vi "main.vi"() -> ()   [LabVIEW 2018]
uses:
  global.vi
  <vilib>/Utility/file.llb/Write Delimited Spreadsheet (string).vi
  <vilib>/Analysis/NI_AALBase.lvlib
panel:
  in  "开始测试":T1
  out "stimulus setup":T2
  in  "字符串":string
  out "二维图片":picture
  out "传声器 1":dbl[](graph)
  out "传声器 2":dbl[](graph)
  out "传声器 3":dbl[](graph)
  out "传声器 4":dbl[](graph)
  in  "阻抗测试绘图数据选择":u16(ring) items=["阻抗Z", "速度V"]
  in  "平滑":dbl(slide) scale=0.0..1.0
  out "速度V":cluster{"f":dbl[], dbl[]}[](graph)
  out "阻抗Z":cluster{dbl[], dbl[]}[](graph)
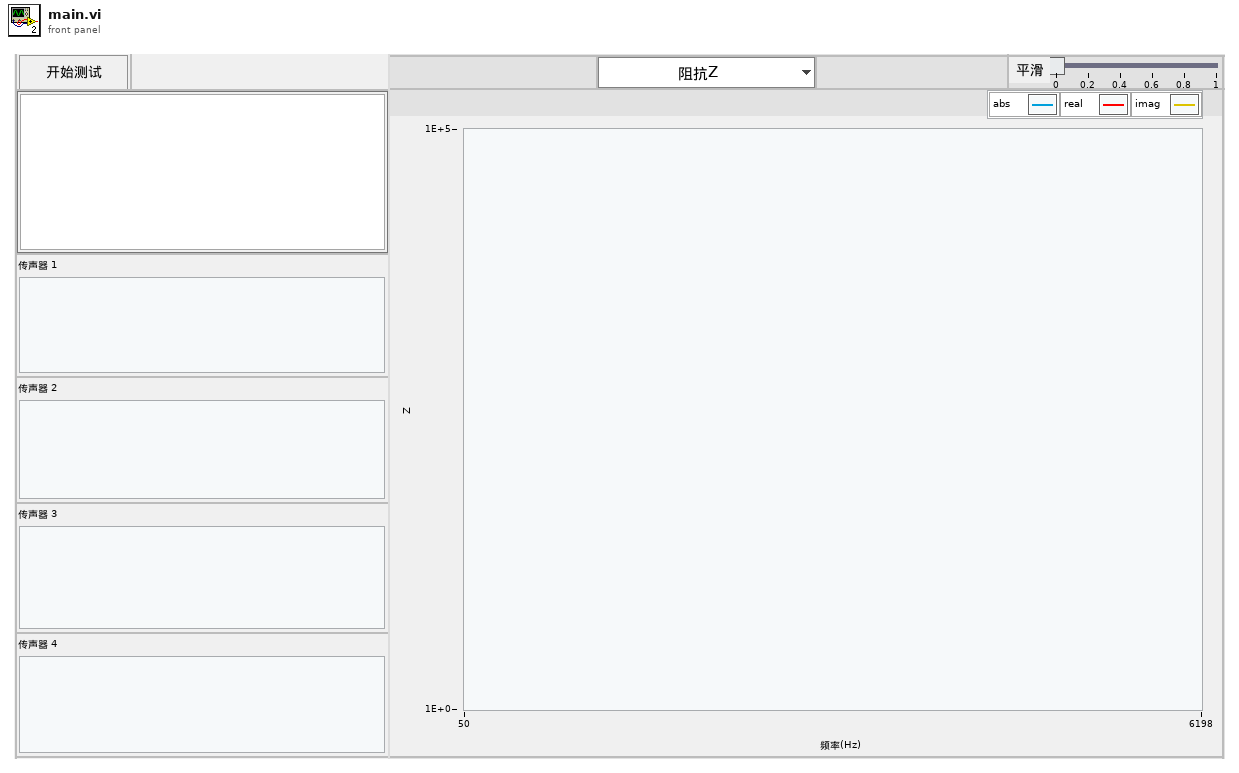
[diagram p1: front panel]
types:
  T1 = typedef "布尔控件.ctl" = bool
  T2 = cluster{"幅值(V)":dbl, "信号时长(s)":dbl, "频率上限(Hz)":dbl, "频率下限(Hz)":dbl}
  T3 = cluster{"f":dbl[], "传输阻抗Z":cdb[], "V":cdb[], "f_V":dbl[]}
  T4 = cluster{"管中温度：":dbl, "阻抗管内径d[mm]：":dbl, "传声器4到样品距离L[mm]：":dbl, "待测样品面积S[mm^2]：":dbl, "mic4灵敏度(V/Pa)：":dbl, "传声器1到样品距离x1[mm]：":dbl, "传声器1到样品距离x2[mm]：":dbl, "传声器1到样品距离x3[mm]：":dbl, "f1":dbl, "f2":dbl, "f3":dbl}
  T5 = enum32{"invalid app kind", "Development System", "Run Time System", "Student Edition", "Embedded LabVIEW", "Evaluation", "Custom"}
  T6 = typedef "LVPoint32TypeDef.ctl" = cluster{"Horizontal":i32, "Vertical":i32}
  T7 = typedef "LVPointDoubleTypeDef.ctl" = cluster{"Cursor X":dbl, "Cursor Y":dbl}
  T8 = typedef "imagedata.ctl" = cluster{"image type":i32, "image depth":i32, "image":u8[], "mask":u8[], "colors":u32[], "Rectangle":cluster{"left":i16, "top":i16, "right":i16, "bottom":i16}}
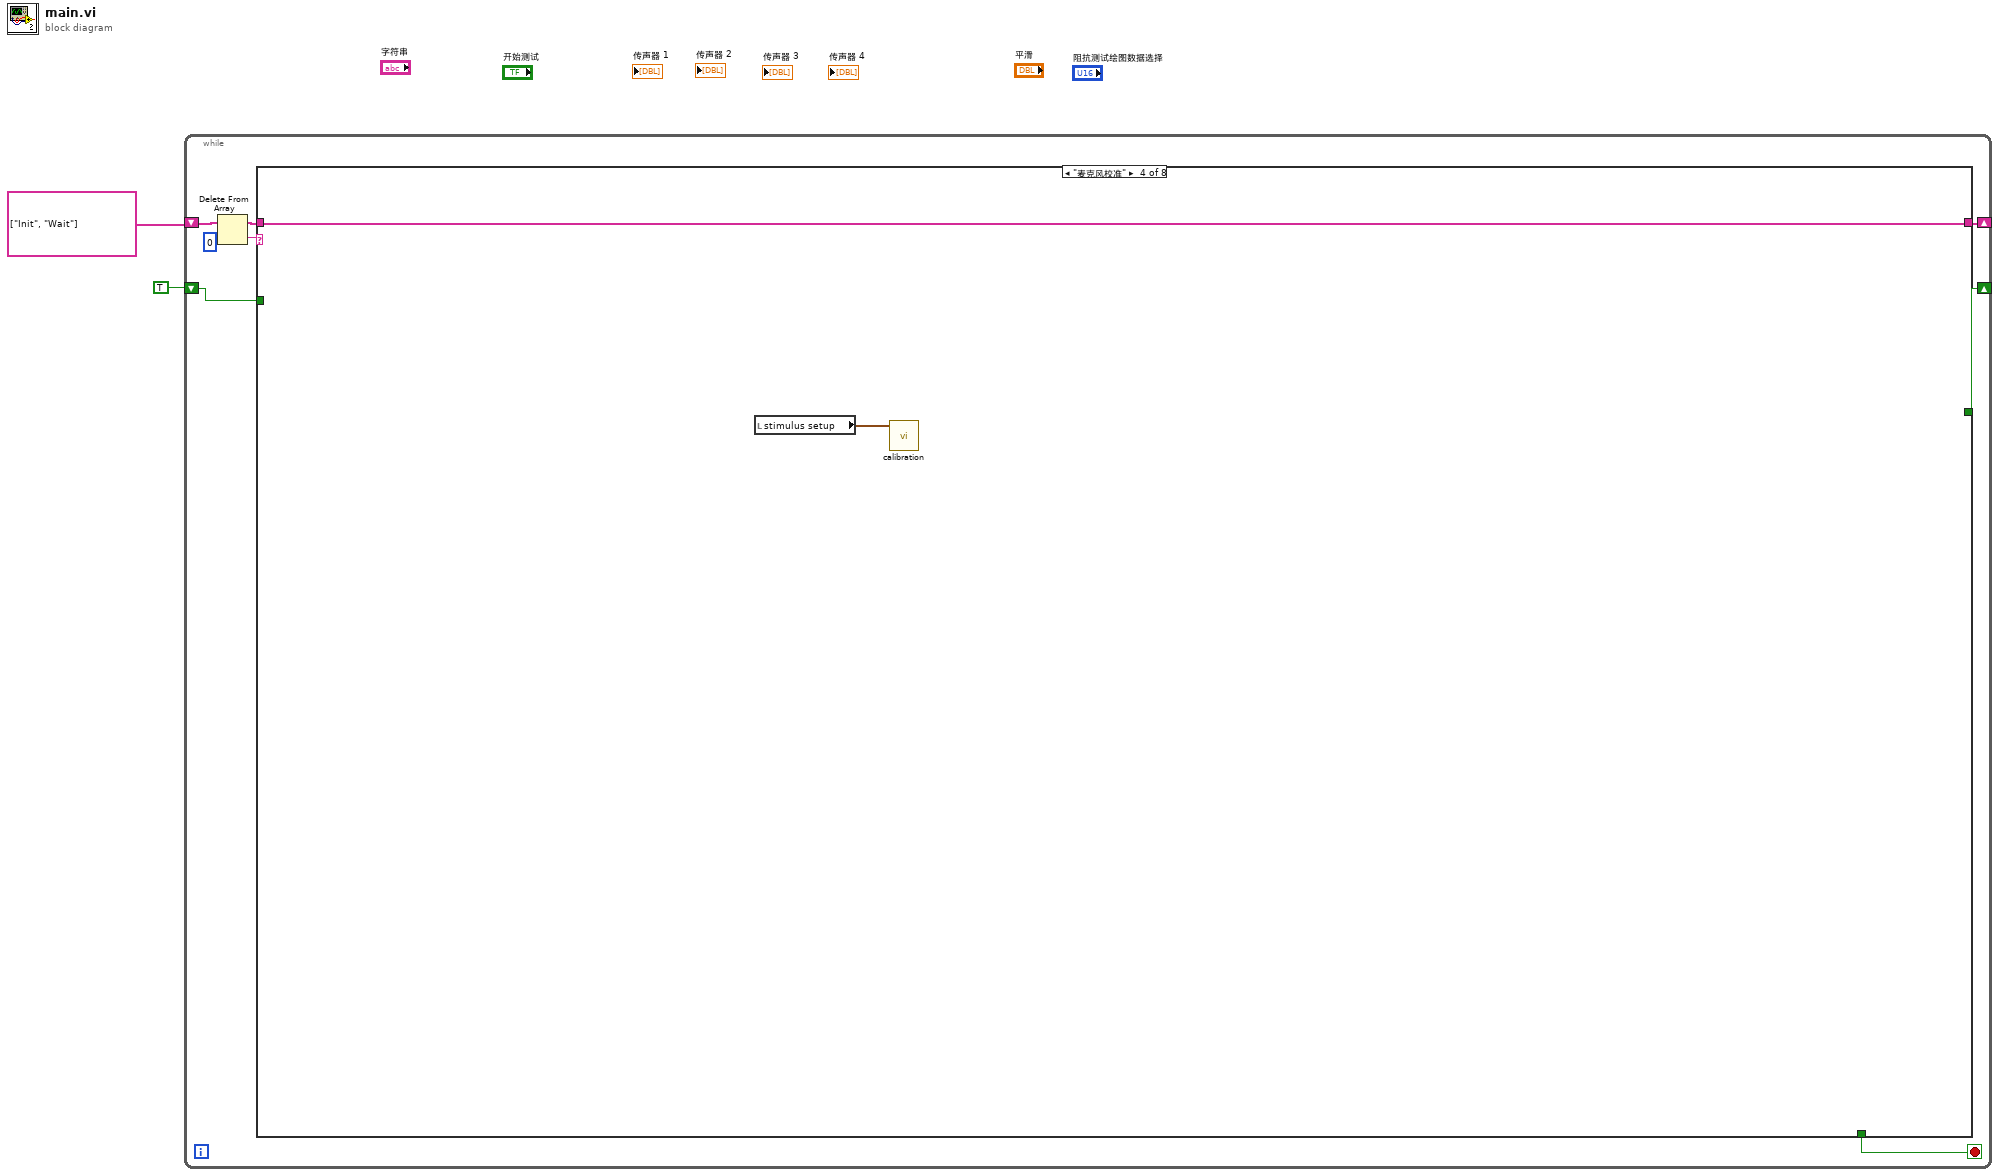
[diagram p0: block diagram]
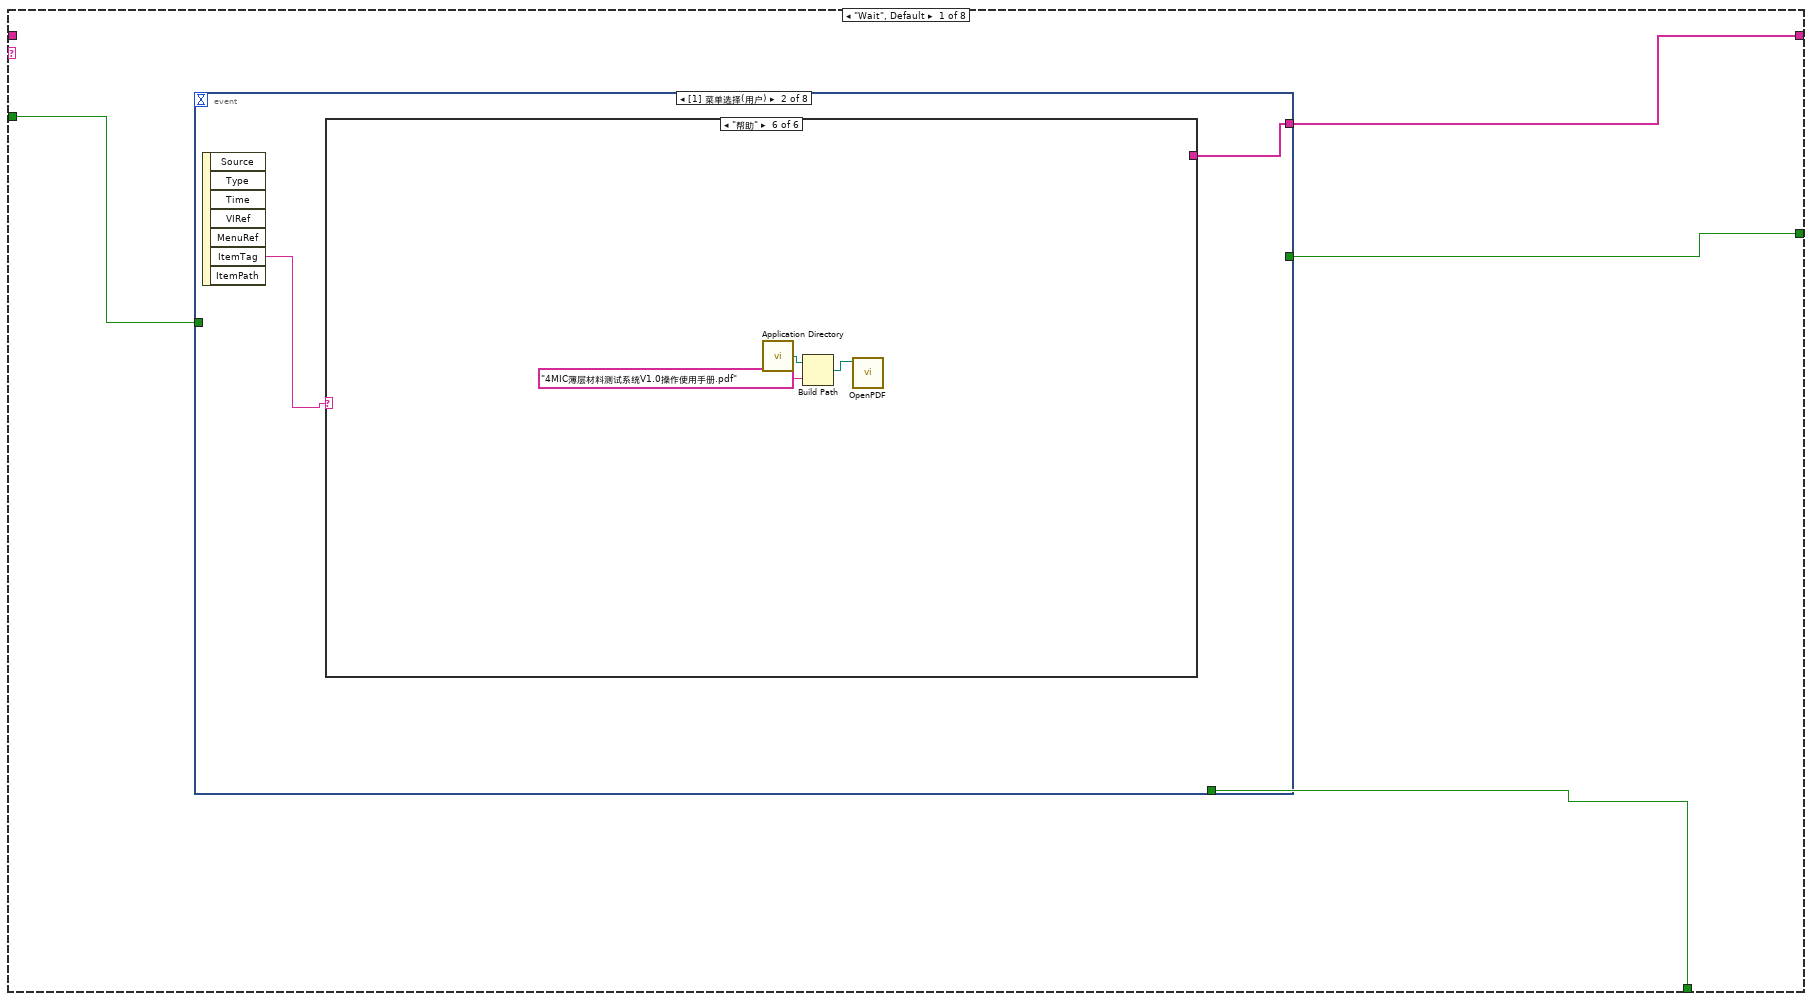
[diagram p2: hidden frame]
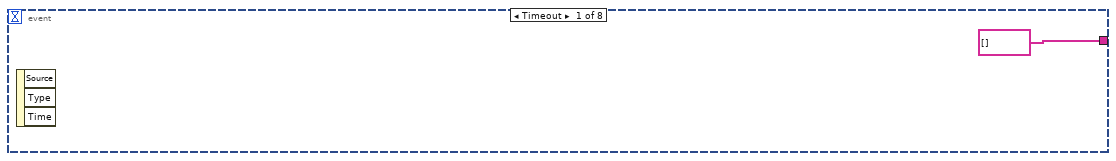
[diagram p3: hidden frame]
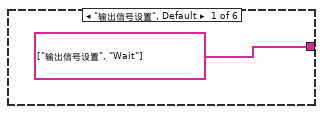
[diagram p4: hidden frame]
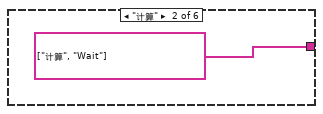
[diagram p5: hidden frame]
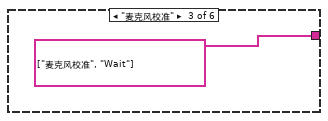
[diagram p6: hidden frame]
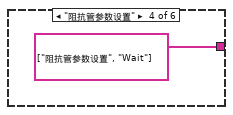
[diagram p7: hidden frame]
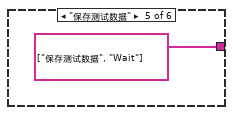
[diagram p8: hidden frame]
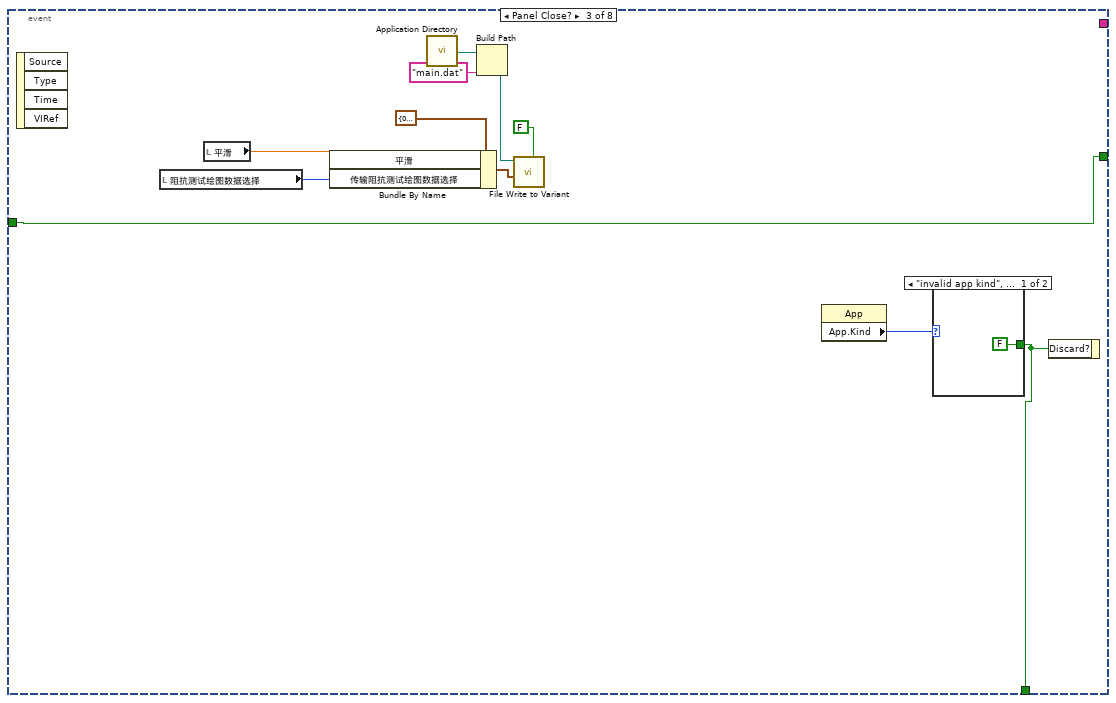
[diagram p9: hidden frame]
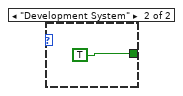
[diagram p10: hidden frame]
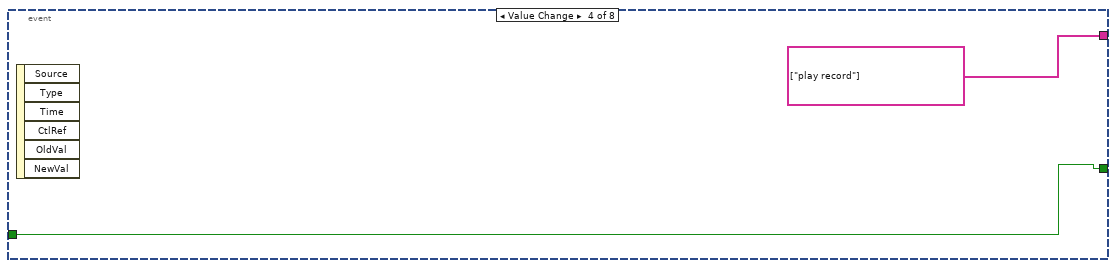
[diagram p11: hidden frame]
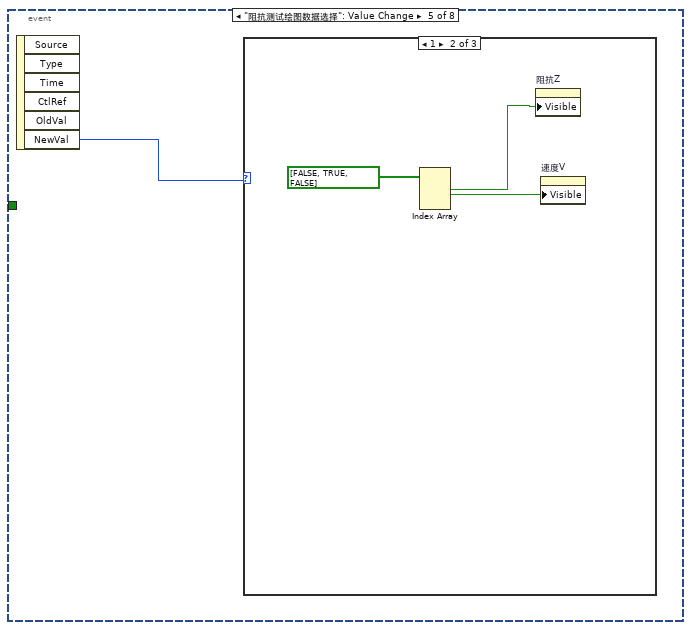
[diagram p12: hidden frame]
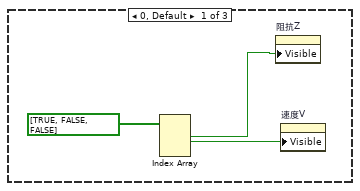
[diagram p13: hidden frame]
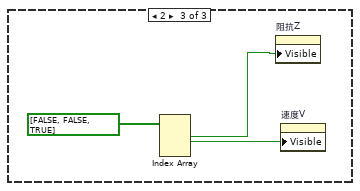
[diagram p14: hidden frame]
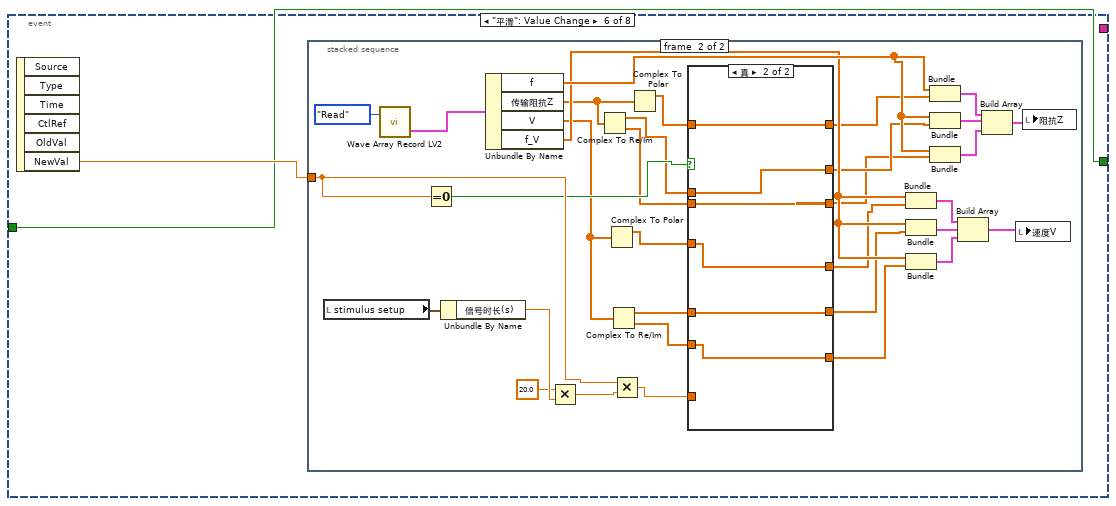
[diagram p15: hidden frame]
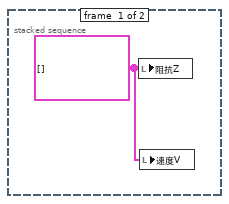
[diagram p16: hidden frame]
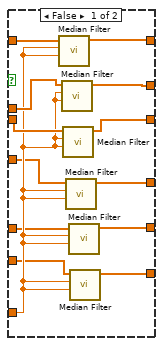
[diagram p17: hidden frame]
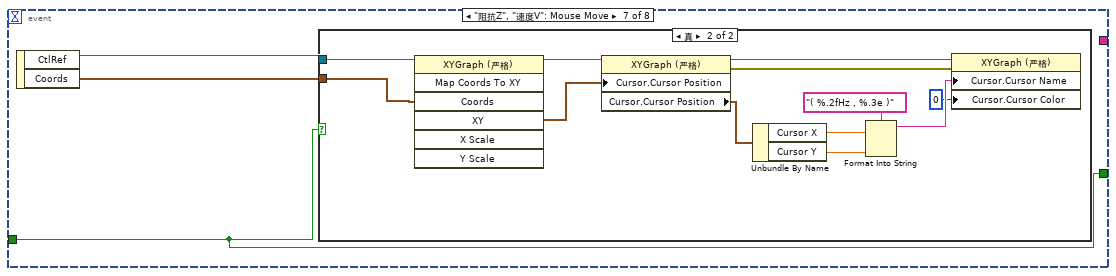
[diagram p18: hidden frame]
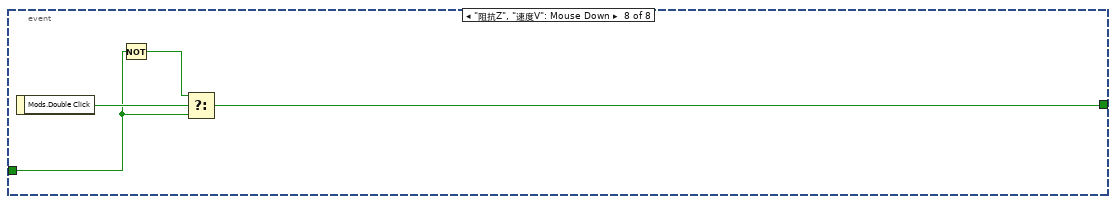
[diagram p20: hidden frame]
diagram:
  n1 = while {
    shift-right: [w6] -> _
    shift-left: string[] ["Init", "Wait"] -> [w10]
    shift-right: [w3] -> _
    shift-left: TRUE ("x") -> [w4]
    stop <- w5 stop-if-true
    n2 = Delete From Array(array=w10, index=0 ("索引")) -> (deleted portion=w8:string, array with subset deleted=w7:string[])  [unwired: 1 in]
    n3 = case shown="\"麦克风校准\"" w8 {
      tunnel: w7 -> [_ w155 w209 w249 w361 w400 w402 w403]
      tunnel: [w14 w155 w208 w249 w361 w400 w402 w403] -> w6
      tunnel: [w13 _ _ _ _ _ _ _] -> w5
      tunnel: w4 -> [w12 _ _ _ _ _ _ _]
      tunnel: [w11 _ _ _ _ _ _ _] -> w3
      frame "Wait", Default {
        n4 = event shown="[1] 菜单选择(用户)" {
          selector: _ -> [_ _ _ _ _ _ _ _]
          dyn-events: _ -> [_ _ _ _ _ _ _ _]
          timeout: _ -> [_ _ _ _ _ _ _ _]
          tunnel: [string[] [] w16 _ string[] ["play record"] _ _ _ _] -> w14
          tunnel: [_ _ w36 _ _ _ _ _] -> w13
          tunnel: w12 -> [_ _ w26 w39 _ w51 w106 w122]
          tunnel: [_ _ w26 w39 _ w51 w106 w121] -> w11
          event Timeout {
            n5 = event-data() -> ()  [unwired: 1 in, 3 out]
          }
          event Menu Selection (User) {
            n6 = event-data() -> ("ItemTag"=w17:string)  [unwired: 1 in, 6 out]
            n7 = case shown="\"帮助\"" w17 {
              tunnel: [string[] ["输出信号设置", "Wait"] string[] ["计算", "Wait"] string[] ["麦克风校准", "Wait"] string[] ["阻抗管参数设置", "Wait"] string[] ["保存测试数据", "Wait"] _] -> w16
              frame "输出信号设置", Default {
              }
              frame "计算" {
              }
              frame "麦克风校准" {
              }
              frame "阻抗管参数设置" {
              }
              frame "保存测试数据" {
              }
              frame "帮助" {
                n8 = call <vilib>:"Application Directory.vi"() -> ("Application Directory"=w25:path)
                n9 = Build Path(base path=w25, name or relative path="4MIC薄层材料测试系统V1.0操作使用手册.pdf" ("名称或相对路径")) -> (appended path=w23:path)
                n10 = call "OpenPDF.vi"("Path"=w23) -> ()  [unwired: 5 in, 2 out]
              }
            }
          }
          event Panel Close? {
            n11 = event-data() -> ()  [unwired: 1 in, 4 out]
            n12 = local read "阻抗测试绘图数据选择"() -> (w32:u16)
            n13 = local read "平滑"() -> (w33:dbl)
            n14 = Bundle By Name(cluster=cluster{"平滑":dbl, "传输阻抗测试绘图数据选择":u16} {"平滑"=0.0, "传输阻抗测试绘图数据选择"=0}, "平滑"=w33, "传输阻抗测试绘图数据选择"=w32) -> (w31:cluster{"平滑":dbl, "传输阻抗测试绘图数据选择":u16})
            n15 = call <vilib>:"Application Directory.vi"() -> ("Application Directory"=w30:path)
            n16 = Build Path(base path=w30, name or relative path="main.dat" ("名称或相对路径")) -> (appended path=w28:path)
            n17 = call "File Write to Variant.vi"("替换提示"=FALSE, "Input Data"=w31, "Path to Write"=w28) -> ()  [unwired: 4 in, 5 out]
            n18 = property class="App"() -> ("App.Kind"=w35:T5)  [unwired: 2 in, 2 out]
            n19 = case shown="\"invalid app kind\", 默认" w35 {
              tunnel: [FALSE ("放弃？") TRUE ("放弃？")] -> w36
              frame "invalid app kind", Default {
              }
              frame "Development System" {
              }
            }
            n20 = event-data("Discard?"=w36) -> ()  [unwired: 1 in, 1 out]
          }
          event Value Change {
            n21 = event-data() -> ()  [unwired: 1 in, 6 out]
          }
          event "阻抗测试绘图数据选择": Value Change {
            n22 = event-data() -> ("NewVal"=w41:u16)  [unwired: 1 in, 5 out]
            n23 = case shown="1" w41 {
              frame 0, Default {
                n24 = Index Array(array=bool[] [TRUE, FALSE, FALSE]) -> (element #1=w43:bool, element #2=w42:bool)  [unwired: 3 in, 1 out]
                n25 = property on="阻抗Z" class="XYGraph (严格)"("Visible"=w43) -> ()  [unwired: 2 in, 2 out]
                n26 = property on="速度V" class="XYGraph (严格)"("Visible"=w42) -> ()  [unwired: 2 in, 2 out]
              }
              frame 1 {
                n27 = Index Array(array=bool[] [FALSE, TRUE, FALSE]) -> (element #1=w46:bool, element #2=w45:bool)  [unwired: 3 in, 1 out]
                n28 = property on="阻抗Z" class="XYGraph (严格)"("Visible"=w46) -> ()  [unwired: 2 in, 2 out]
                n29 = property on="速度V" class="XYGraph (严格)"("Visible"=w45) -> ()  [unwired: 2 in, 2 out]
              }
              frame 2 {
                n30 = Index Array(array=bool[] [FALSE, FALSE, TRUE]) -> (element #1=w49:bool, element #2=w48:bool)  [unwired: 3 in, 1 out]
                n31 = property on="阻抗Z" class="XYGraph (严格)"("Visible"=w49) -> ()  [unwired: 2 in, 2 out]
                n32 = property on="速度V" class="XYGraph (严格)"("Visible"=w48) -> ()  [unwired: 2 in, 2 out]
              }
            }
          }
          event "平滑": Value Change {
            n33 = event-data() -> ("NewVal"=w52:dbl)  [unwired: 1 in, 5 out]
            n34 = stacked-sequence {
              tunnel: w52 -> [_ w80]
              frame #0 {
                w53 = cluster{dbl[], dbl[]}[] [] ("阻抗Z")
                n35 = local write "阻抗Z"(w53) -> ()
                n36 = local write "速度V"(w53) -> ()
              }
              frame #1 {
                n37 = local read "stimulus setup"() -> (w86:T2)
                n38 = call "Wave Array Record LV2.vi"("W / R"=enum16{"Write", "Read"}."Read") -> ("吸声测试结果Out"=w82:T3)  [unwired: 2 in]
                n39 = Equal To 0?(x=w80) -> (x = 0?=w73:bool)
                n40 = Unbundle By Name(w86) -> ("信号时长(s)"=w85:dbl)
                n41 = Unbundle By Name(w82) -> ("f"=w79:dbl[], "传输阻抗Z"=w72:cdb[], "V"=w59:cdb[], "f_V"=w74:dbl[])
                n42 = Multiply(x=20.0, y=w85) -> (x*y=w81:dbl)
                n43 = Complex To Re/Im(x + iy=w72) -> (x=w70:dbl[], y=w69:dbl[])
                n44 = Complex To Polar(r * e^(i*theta)=w59) -> (r=w60:dbl[])  [unwired: 1 out]
                n45 = Complex To Re/Im(x + iy=w59) -> (x=w58:dbl[], y=w55:dbl[])
                n46 = Multiply(x=w80, y=w81) -> (x*y=w68:dbl)
                n47 = Complex To Polar(r * e^(i*theta)=w72) -> (r=w71:dbl[])  [unwired: 1 out]
                n48 = case shown="真" w73 {
                  tunnel: w70 -> [w97 w104]
                  tunnel: w69 -> [w95 w103]
                  tunnel: w71 -> [w99 w105]
                  tunnel: [w98 w105] -> w67
                  tunnel: [w96 w104] -> w66
                  tunnel: [w94 w103] -> w65
                  tunnel: w68 -> [w93 _]
                  tunnel: w60 -> [w92 w102]
                  tunnel: [w91 w102] -> w57
                  tunnel: w58 -> [w90 w101]
                  tunnel: [w89 w101] -> w56
                  tunnel: w55 -> [w88 w100]
                  tunnel: [w87 w100] -> w54
                  frame False {
                    n49 = call <vilib>:"Median Filter.vi"("right rank"=w93, "left rank"=w93, "X"=w99) -> ("Filtered X"=w98:dbl[])  [unwired: 7 in, 1 out]
                    n50 = call <vilib>:"Median Filter.vi"("right rank"=w93, "left rank"=w93, "X"=w97) -> ("Filtered X"=w96:dbl[])  [unwired: 7 in, 1 out]
                    n51 = call <vilib>:"Median Filter.vi"("right rank"=w93, "left rank"=w93, "X"=w95) -> ("Filtered X"=w94:dbl[])  [unwired: 7 in, 1 out]
                    n52 = call <vilib>:"Median Filter.vi"("right rank"=w93, "left rank"=w93, "X"=w92) -> ("Filtered X"=w91:dbl[])  [unwired: 7 in, 1 out]
                    n53 = call <vilib>:"Median Filter.vi"("right rank"=w93, "left rank"=w93, "X"=w90) -> ("Filtered X"=w89:dbl[])  [unwired: 7 in, 1 out]
                    n54 = call <vilib>:"Median Filter.vi"("right rank"=w93, "left rank"=w93, "X"=w88) -> ("Filtered X"=w87:dbl[])  [unwired: 7 in, 1 out]
                  }
                  frame True {
                  }
                }
                n55 = Bundle("f_V"=w74, "Filtered X"=w57) -> (w75:cluster{"f_V":dbl[], "Filtered X":dbl[]})  [unwired: 1 in]
                n56 = Bundle("f_V"=w74, "Filtered X"=w56) -> (w76:cluster{"f_V":dbl[], "Filtered X":dbl[]})  [unwired: 1 in]
                n57 = Bundle("f_V"=w74, "Filtered X"=w54) -> (w77:cluster{"f_V":dbl[], "Filtered X":dbl[]})  [unwired: 1 in]
                n58 = Bundle("f"=w79, "Filtered X"=w67) -> (w78:cluster{"f":dbl[], "Filtered X":dbl[]})  [unwired: 1 in]
                n59 = Bundle("f"=w79, "Filtered X"=w66) -> (w64:cluster{"f":dbl[], "Filtered X":dbl[]})  [unwired: 1 in]
                n60 = Bundle("f"=w79, "Filtered X"=w65) -> (w63:cluster{"f":dbl[], "Filtered X":dbl[]})  [unwired: 1 in]
                n61 = Build Array(w75, w76, w77) -> (w61:cluster{"f_V":dbl[], "Filtered X":dbl[]}[])
                n62 = Build Array(w78, w64, w63) -> (w62:cluster{"f":dbl[], "Filtered X":dbl[]}[])
                n63 = local write "速度V"(w61) -> ()
                n64 = local write "阻抗Z"(w62) -> ()
              }
            }
          }
          event "阻抗Z", "速度V": Mouse Move {
            n65 = event-data() -> ("CtlRef"=w108:refnum<vi>, "Coords"=w107:T6)  [unwired: 1 in]
            n66 = case shown="真" w106 {
              tunnel: w108 -> [_ w120]
              tunnel: w107 -> [_ w117]
              frame False {
              }
              frame True {
                n67 = invoke class="XYGraph (严格)" method="Map Coords To XY"(reference=w120, "Coords"=w117) -> (reference out=w119:refnum<vi>, "XY"=w118:cluster{"X":dbl, "Y":dbl})  [unwired: 5 in, 5 out]
                n68 = property class="XYGraph (严格)"(reference=w119, "Cursor.Cursor Position"=w118) -> (reference out=w116:refnum<vi>, error out=w115:errorcluster, "Cursor.Cursor Position"=w114:T7)  [unwired: 1 in]
                n69 = Unbundle By Name(w114) -> ("Cursor X"=w112:dbl, "Cursor Y"=w111:dbl)
                n70 = Format Into String(format string="( %.2fHz , %.3e )" ("格式字符串"), w112, w111) -> (resulting string=w110:string)  [unwired: 2 in, 1 out]
                n71 = property class="XYGraph (严格)"(reference=w116, error in=w115, "Cursor.Cursor Name"=w110, "Cursor.Cursor Color"=u32 0 ("游标.游标颜色")) -> ()  [unwired: 2 out]
              }
            }
          }
          event "阻抗Z", "速度V": Mouse Down {
            n72 = event-data() -> ("Mods.Double Click"=w124:bool)  [unwired: 1 in]
            n73 = Not(x=w122) -> (.not. x?=w123:bool)
            n74 = Select(t=w123, s=w124, f=w122) -> (s? t:f=w121:bool)
          }
        }
      }
      frame "Init" {
        n75 = call <vilib>:"Application Directory.vi"() -> ("Application Directory"=w148:path)
        n76 = call <vilib>:"Application Directory.vi"() -> ("Application Directory"=w135:path)
        n77 = Build Path(base path=w148, name or relative path="main.dat" ("名称或相对路径")) -> (appended path=w146:path)
        n78 = property on="开始测试" class="Bool (严格)"("Value"=T1 FALSE ("开始测试"), "Visible"=TRUE ("可见")) -> ()  [unwired: 2 in, 2 out]
        n79 = property on="字符串" class="Str"("Visible"=FALSE ("可见"), "Value"="测试中······" ("字符串"), "Text.TextColor"=u32 32639, "Text.FontSize"=u32 30 ("文本.字体:字号")) -> ()  [unwired: 2 in, 2 out]
        n80 = call "File Read Binary File.vi"("file path"=w146) -> ("error Output"=w142:errorcluster, "Variant Output"=w145:variant)  [unwired: 8 in, 1 out]
        n81 = Build Path(base path=w135, name or relative path="stimulus.dat" ("名称或相对路径")) -> (appended path=w139:path)
        n82 = case shown="无错误" w142 {
          tunnel: w145 -> [w161 _]
          tunnel: [w160 _] -> w144
          frame No Error {
            n83 = Variant To Data(type=cluster{"平滑":dbl, "阻抗测试绘图数据选择":u16} {"平滑"=0.0, "阻抗测试绘图数据选择"=0}, Variant=w161) -> (data=w160:cluster{"平滑":dbl, "阻抗测试绘图数据选择":u16})  [unwired: 1 in, 1 out]
          }
          frame Error {
          }
        }
        n84 = call "File Read Binary File.vi"("file path"=w139) -> ("error Output"=w140:errorcluster, "Variant Output"=w141:variant)  [unwired: 8 in, 1 out]
        n85 = case shown="无错误" w140 {
          tunnel: w141 -> [w158 _]
          tunnel: [w156 _] -> w137
          frame No Error {
            n86 = Variant To Data(type=T2 {"幅值(V)"=1.0, "信号时长(s)"=3.0, "频率上限(Hz)"=20000.0, "频率下限(Hz)"=10.0} ("stimulus setup"), Variant=w158) -> (data=w156:T2)  [unwired: 1 in, 1 out]
          }
          frame Error {
          }
        }
        n87 = local write "stimulus setup"(w137) -> ()
        n88 = Unbundle By Name(w144) -> ("平滑"=w143:dbl, "阻抗测试绘图数据选择"=w136:u16)
        n89 = property on="平滑" class="Slide (严格)"("Val(Sgnl)"=w143) -> ()  [unwired: 2 in, 2 out]
        n90 = call <vilib>:"Application Directory.vi"() -> ("Application Directory"=w134:path)
        n91 = Build Path(base path=w134, name or relative path="示意图.png" ("t")) -> (appended path=w154:path)
        n92 = property on="阻抗测试绘图数据选择" class="Ring (严格)"("Val(Sgnl)"=w136) -> ()  [unwired: 2 in, 2 out]
        n93 = call <vilib>:"Read PNG File.vi"("path to PNG file"=w154) -> ("image data"=w153:T8)  [unwired: 8 in, 2 out]
        n94 = call <vilib>:"Draw Flattened Pixmap.vi"("image data"=w153) -> ("new picture"=→"二维图片":picture)  [unwired: 8 in]
        n95 = global write "global.vi" "Format"(cluster{"Rate":i32, "Bits":i32, "Channels":u32} {"Rate"=44100, "Bits"=32, "Channels"=4} ("Format")) -> ()
        n96 = property on="阻抗Z" class="XYGraph (严格)"("Visible"=TRUE ("可见")) -> ()  [unwired: 2 in, 2 out]
        n97 = property on="速度V" class="XYGraph (严格)"("Visible"=FALSE ("可见")) -> ()  [unwired: 2 in, 2 out]
        n98 = property on="阻抗测试绘图数据选择" class="Ring (严格)"("Visible"=TRUE ("可见"), "Strings []"=string[] ["阻抗Z", "速度V"] ("字符串[]")) -> ()  [unwired: 2 in, 2 out]
      }
      frame "play record" {
        n99 = local read "stimulus setup"() -> (w210:T2)
        n100 = Unbundle By Name(w210) -> ("幅值(V)"=w217:dbl, "信号时长(s)"=w214:dbl, "频率上限(Hz)"=w216:dbl, "频率下限(Hz)"=w215:dbl)
        n101 = global read "global.vi" "Format"() -> (w212:cluster{"Rate":i32, "Bits":i32, "Channels":u32})
        n102 = property on="开始测试" class="Bool (严格)"("Visible"=FALSE ("可见")) -> (error out=w195:errorcluster)  [unwired: 2 in, 1 out]
        n103 = Unbundle By Name(w212) -> ("Rate"=w211:i32)
        n104 = property on="字符串" class="Str"(error in=w195, "Visible"=TRUE ("可见"), "Value"="测试中······" ("字符串"), "Text.FontColor"=u32 32639, "Text.FontSize"=u32 30 ("文本.字体:字号")) -> (error out=w194:errorcluster)  [unwired: 1 in, 1 out]
        n105 = call "stimulus.vi"("error play 2"=w194, "幅值(V)"=w217, "stop frequency [Hz]"=w216, "start frequency [Hz]"=w215, "信号时长"=w214, "Format"=w212) -> ("error play 3"=w197:errorcluster, "data length"=w219:i32, "Output data"=w220:i32[][])  [unwired: 2 in, 1 out]
        n106 = Reciprocal(x=w211) -> (1/x=w174:dbl)
        n107 = call "asio_out_in.vi"("error play 4"=w197, "信号时长"=w214, "Format"=w212, "card #"=u32 0, "data_length"=w219, "output data"=w220) -> ("error play 2"=w193:errorcluster, "MIC_Data_IN"=w213:dbl[][])  [unwired: 3 in, 1 out]
        n108 = case shown="无错误" w193 {
          tunnel: w193 -> [w223 w235]
          frame No Error {
            n109 = property on="字符串" class="Str"(error in=w223, "Visible"=FALSE ("可见")) -> (error out=w222:errorcluster)  [unwired: 1 in, 1 out]
            n110 = property on="开始测试" class="Bool (严格)"(error in=w222, "Value"=T1 FALSE ("开始测试"), "Visible"=TRUE ("可见")) -> ()  [unwired: 1 in, 2 out]
          }
          frame Error {
            n111 = Unbundle By Name(w235) -> ("code"=w230:i32, "source"=w227:string)
            n112 = Number To Decimal String(number=w230) -> (decimal integer string=w229:string)  [unwired: 1 in]
            n113 = Concatenate Strings("错误代码：" ("字符串"), w229, "\n", w227) -> (w226:string)
            n114 = call "WriteLog.vi"("String"=w226) -> ()  [unwired: 2 in]
            n115 = case shown="默认" w230 {
              tunnel: [w236 w240 w244] -> w234
              frame -1098 {
                n116 = property on="字符串" class="Str"("Value"="测试异常······\n未检测到声卡" ("字符串"), "Text.TextColor"=u32 16711680, "Text.FontSize"=u32 16 ("文本.字体:字号")) -> (error out=w236:errorcluster)  [unwired: 2 in, 1 out]
              }
              frame -1101 {
                n117 = property on="字符串" class="Str"("Value"="测试异常······输出信号设置错误" ("字符串"), "Text.TextColor"=u32 16711680, "Text.FontSize"=u32 16 ("文本.字体:字号")) -> (error out=w240:errorcluster)  [unwired: 2 in, 1 out]
              }
              frame Default {
                n118 = property on="字符串" class="Str"("Value"="测试异常······\n音频播放采集错误" ("字符串"), "Text.TextColor"=u32 16711680, "Text.FontSize"=u32 16 ("文本.字体:字号")) -> (error out=w244:errorcluster)  [unwired: 2 in, 1 out]
              }
            }
            n119 = property on="开始测试" class="Bool (严格)"(error in=w234, "Value"=T1 FALSE ("开始测试"), "Visible"=TRUE ("可见")) -> ()  [unwired: 1 in, 2 out]
          }
        }
        n120 = Index Array(array=w213, index (row) #1=0 ("索引 (行)"), index (row) #2=1 ("索引 (行)"), index (row) #3=2 ("索引 (行)"), index (row) #4=3 ("索引 (行)")) -> (element #1=w187:dbl[], element #2=w169:dbl[], element #3=w168:dbl[], element #4=w167:dbl[])  [unwired: 4 in]
        n121 = Absolute Value(x=w168) -> (abs(x)=w171:dbl[])
        n122 = Absolute Value(x=w187) -> (abs(x)=w186:dbl[])
        n123 = Absolute Value(x=w167) -> (abs(x)=w172:dbl[])
        n124 = Absolute Value(x=w169) -> (abs(x)=w185:dbl[])
        n125 = Bundle By Name("Y"=w187, "dt"=w174) -> (w200:waveform(dbl))  [unwired: 1 in]
        n126 = Bundle By Name("Y"=w169, "dt"=w174) -> (w199:waveform(dbl))  [unwired: 1 in]
        n127 = Bundle By Name("Y"=w168, "dt"=w174) -> (w180:waveform(dbl))  [unwired: 1 in]
        n128 = Bundle By Name("Y"=w167, "dt"=w174) -> (w175:waveform(dbl))  [unwired: 1 in]
        n129 = Array Max & Min(array=w172) -> (max value=w170:dbl)  [unwired: 3 out]
        n130 = Array Max & Min(array=w185) -> (max value=w188:dbl)  [unwired: 3 out]
        n131 = Array Max & Min(array=w171) -> (max value=w162:dbl)  [unwired: 3 out]
        n132 = Array Max & Min(array=w186) -> (max value=w189:dbl)  [unwired: 3 out]
        n133 = Max & Min(x=w162, y=w170) -> (max(x,y)=w165:dbl)  [unwired: 1 out]
        n134 = Max & Min(x=w189, y=w188) -> (max(x,y)=w166:dbl)  [unwired: 1 out]
        n135 = Max & Min(x=w166, y=w165) -> (max(x,y)=w164:dbl)  [unwired: 1 out]
        n136 = Insert Into Array(array=w209, new element=string[] ["计算", "Wait"]) -> (w208:string[])  [unwired: 1 in]
        n137 = local write "传声器 2"(w199) -> ()
        n138 = local write "传声器 3"(w180) -> ()
        n139 = local write "传声器 4"(w175) -> ()
        n140 = local write "传声器 1"(w200) -> ()
        n141 = Multiply(x=w164, y=1.1) -> (x*y=w163:dbl)
        n142 = call "save_wav_as_txt.vi"("文件夹名"="！采集", "txt名"="MIC1.txt", "wav"=w187) -> ()  [unwired: 9 in]
        n143 = Negate(x=w163) -> (-x=w173:dbl)
        n144 = Negate(x=w163) -> (-x=w184:dbl)
        n145 = call "save_wav_as_txt.vi"("文件夹名"="！采集", "txt名"="MIC2.txt", "wav"=w169) -> ()  [unwired: 9 in]
        n146 = call "save_wav_as_txt.vi"("文件夹名"="！采集", "txt名"="MIC3.txt", "wav"=w168) -> ()  [unwired: 9 in]
        n147 = property on="传声器 3" class="WFGraph (严格)"("YScale.Maximum"=w163, "YScale.Minimum"=w173) -> ()  [unwired: 2 in, 2 out]
        n148 = property on="传声器 1" class="WFGraph (严格)"("YScale.Maximum"=w163, "YScale.Minimum"=w184) -> ()  [unwired: 2 in, 2 out]
        n149 = property on="传声器 4" class="WFGraph (严格)"("YScale.Maximum"=w163, "YScale.Minimum"=w173) -> ()  [unwired: 2 in, 2 out]
        n150 = call "save_wav_as_txt.vi"("文件夹名"="！采集", "txt名"="MIC4.txt", "wav"=w167) -> ()  [unwired: 9 in]
        n151 = property on="传声器 2" class="WFGraph (严格)"("YScale.Maximum"=w163, "YScale.Minimum"=w184) -> ()  [unwired: 2 in, 2 out]
      }
      frame "麦克风校准" {
        n152 = local read "stimulus setup"() -> (w248:T2)
        n153 = call "calibration.vi"("输入簇"=w248) -> ()  [unwired: 11 in]
      }
      frame "计算" {
        w344 = 50.0 ("X标尺.范围:最小值")
        w312 = 1000.0 ("y")
        w357 = u32 16777222
        w347 = u8 1 ("X标尺.映射模式")
        w348 = u8 1 ("X标尺.映射模式")
        # "H43"
        # "H23"
        # "H13"
        n154 = call <vilib>:"Application Directory.vi"() -> ("Application Directory"=w354:path)
        n155 = global read "global.vi" "Format"() -> (w370:cluster{"Rate":i32, "Bits":i32, "Channels":u32})
        n156 = Build Path(base path=w354, name or relative path="parameter.dat" ("名称或相对路径")) -> (appended path=w366:path)
        n157 = call "File Read Binary File.vi"("file path"=w366) -> ("error Output"=w356:errorcluster, "Variant Output"=w367:variant)  [unwired: 8 in, 1 out]
        n158 = case shown="无错误" w356 {
          tunnel: w367 -> [w398 _]
          tunnel: [w397 _] -> w364
          frame No Error {
            n159 = Variant To Data(type=T4 {"管中温度："=22.0, "阻抗管内径d[mm]："=0.2, "传声器4到样品距离L[mm]："=0.025, "待测样品面积S[mm^2]："=0.15, "mic4灵敏度(V/Pa)："=0.0, "传声器1到样品距离x1[mm]："=0.0, "传声器1到样品距离x2[mm]："=0.0, "传声器1到样品距离x3[mm]："=0.0, "f1"=0.0, "f2"=0.0, "f3"=0.0}, Variant=w398) -> (data=w397:T4)  [unwired: 1 in, 1 out]
          }
          frame Error {
            n160 = One Button Dialog(message="先设置阻抗管参数" ("消息")) -> ()  [unwired: 1 in, 1 out]
          }
        }
        n161 = call "read_wav_from_txt.vi"("名称或相对路径"="！校准\\MIC1.txt" ("文件夹名")) -> ("error out"=w339:errorcluster, "wav"=w327:dbl[])  [unwired: 9 in]
        n162 = call "read_wav_from_txt.vi"("名称或相对路径"="！校准\\MIC2.txt" ("文件夹名")) -> ("error out"=w338:errorcluster, "wav"=w326:dbl[])  [unwired: 9 in]
        n163 = Unbundle By Name(w370) -> ("Rate"=w293:i32)
        n164 = call "read_wav_from_txt.vi"("名称或相对路径"="！校准\\MIC3.txt" ("文件夹名")) -> ("error out"=w336:errorcluster, "wav"=w325:dbl[])  [unwired: 9 in]
        n165 = call "read_wav_from_txt.vi"("名称或相对路径"="！校准\\MIC4.txt" ("文件夹名")) -> ("error out"=w337:errorcluster, "wav"=w292:dbl[])  [unwired: 9 in]
        n166 = call "read_wav_from_txt.vi"("名称或相对路径"="！采集\\MIC1.txt" ("文件夹名")) -> ("wav"=w330:dbl[])  [unwired: 9 in, 1 out]
        n167 = call "read_wav_from_txt.vi"("名称或相对路径"="！采集\\MIC3.txt" ("文件夹名")) -> ("wav"=w328:dbl[])  [unwired: 9 in, 1 out]
        n168 = call "read_wav_from_txt.vi"("名称或相对路径"="！采集\\MIC2.txt" ("文件夹名")) -> ("wav"=w329:dbl[])  [unwired: 9 in, 1 out]
        n169 = call "read_wav_from_txt.vi"("名称或相对路径"="！采集\\MIC4.txt" ("文件夹名")) -> ("wav"=w253:dbl[])  [unwired: 9 in, 1 out]
        n170 = Unbundle By Name(w336) -> ("status"=w333:bool)
        n171 = Unbundle By Name(w339) -> ("status"=w335:bool)
        n172 = Unbundle By Name(w337) -> ("status"=w332:bool)
        n173 = Unbundle By Name(w338) -> ("status"=w334:bool)
        n174 = Unbundle By Name(w364) -> ("管中温度："=w363:dbl, "阻抗管内径d[mm]："=w308:dbl, "传声器4到样品距离L[mm]："=w294:dbl, "待测样品面积S[mm^2]："=w309:dbl, "mic4灵敏度(V/Pa)："=w290:dbl, "传声器1到样品距离x1[mm]："=w314:dbl, "传声器1到样品距离x2[mm]："=w316:dbl, "传声器1到样品距离x3[mm]："=w318:dbl, "f1"=w252:dbl, "f2"=w251:dbl, "f3"=w250:dbl)
        n175 = Compound Arithmetic op=OR(w335, w334, w333, w332) -> (w331:bool)
        n176 = call "tfH12.vi"("Resp1"=w330, "采样率"=w293, "Resp2"=w328) -> ("ff"=w301:dbl[], "H12"=w355:cdb[])  [unwired: 3 in]
        n177 = call "tfH12.vi"("Resp1"=w329, "采样率"=w293, "Resp2"=w328) -> ("H12"=w324:cdb[])  [unwired: 3 in, 1 out]
        n178 = call "tfH12.vi"("Resp1"=w253, "采样率"=w293, "Resp2"=w328) -> ("H12"=w322:cdb[])  [unwired: 3 in, 1 out]
        n179 = call "tfH12.vi"("Resp1"=w327, "采样率"=w293, "Resp2"=w325) -> ("H12"=w351:cdb[])  [unwired: 3 in, 1 out]
        n180 = call "tfH12.vi"("Resp1"=w326, "采样率"=w293, "Resp2"=w325) -> ("H12"=w323:cdb[])  [unwired: 3 in, 1 out]
        n181 = call "tfH12.vi"("Resp1"=w292, "采样率"=w293, "Resp2"=w325) -> ("H12"=w321:cdb[])  [unwired: 3 in, 1 out]
        n182 = case shown="真" w331 {
          frame False {
          }
          frame True {
            n183 = One Button Dialog(message="校准文件错误" ("消息")) -> ()  [unwired: 1 in, 1 out]
          }
        }
        n184 = Divide(x=w355, y=w351) -> (x/y=w320:cdb[])
        n185 = Divide(x=w324, y=w323) -> (x/y=w319:cdb[])
        n186 = Divide(x=w322, y=w321) -> (x/y=w306:cdb[])
        n187 = Divide(x=w318, y=w312) -> (x/y=w317:dbl)
        n188 = Divide(x=w308, y=w312) -> (x/y=w291:dbl)
        n189 = Divide(x=w294, y=w312) -> (x/y=w307:dbl)
        n190 = call "基本参数计算.vi"("temp实际摄氏温度"=w363, "atm/kPa"=101.0) -> ("Z0空气的特性阻抗"=w295:dbl, "考虑温度实际声速c0"=w289:dbl)  [unwired: 7 in, 1 out]
        n191 = Divide(x=w316, y=w312) -> (x/y=w315:dbl)
        n192 = Divide(x=w314, y=w312) -> (x/y=w313:dbl)
        n193 = call "计算修正传输波数k.vi"("f"=w301, "c0"=w289, "dia_tube(m)"=w291) -> ("k"=w305:cdb[])  [unwired: 8 in]
        n194 = call "计算反射系数r.vi"("x3"=w317, "x1"=w313, "H13"=w320, "k"=w305) -> ("r complex"=w311:cdb[])  [unwired: 7 in]
        n195 = call "S_factor.vi"("管内径[mm]"=w308, "待测样品面积[mm^2]"=w309) -> ("S_factor"=w288:dbl)  [unwired: 9 in]
        n196 = call "计算反射系数r.vi"("x3"=w317, "x1"=w315, "H13"=w319, "k"=w305) -> ("r complex"=w310:cdb[])  [unwired: 7 in]
        n197 = property on="速度V" class="XYGraph (严格)"("XScale.Maximum"=w250, "XScale.Minimum"=w344, "XScale.Mapping Mode"=w347, "Plot.Plot Color"=w357, "YScale.Mapping Mode"=w347, "YScale.Maximum"=10.0 ("Y标尺.范围:最大值"), "YScale.Minimum"=1e-09 ("Y标尺.范围:最小值")) -> ()  [unwired: 2 in, 2 out]
        n198 = call "计算中高频Z.vi"("特性阻抗Z0"=w295, "r"=w311, "x3"=w317, "factor"=w288, "L"=w307, "H43"=w306, "k"=w305) -> ("Z中高频"=w304:cdb[])  [unwired: 8 in]
        n199 = call "计算中高频Z.vi"("特性阻抗Z0"=w295, "r"=w310, "x3"=w317, "factor"=w288, "L"=w307, "H43"=w306, "k"=w305) -> ("Z中高频"=w303:cdb[])  [unwired: 8 in]
        n200 = call "计算低频Z.vi"("特性阻抗Z0"=w295, "factor"=w288, "L"=w307, "H43"=w306, "k"=w305) -> ("Z低频"=w302:cdb[])  [unwired: 10 in]
        n201 = call "calculate_v.vi"("Z0"=w295, "mic4灵敏度Sen(V/Pa)"=w290, "S_factor"=w288, "L[mm]"=w294, "Rate"=w293, "mic4"=w253, "dia_tube(m)"=w291, "c0"=w289) -> ("V"=w264:cdb[], "f"=w281:dbl[])  [unwired: 6 in]
        n202 = local read "stimulus setup"() -> (w359:T2)
        n203 = Unbundle By Name(w359) -> ("信号时长(s)"=w358:dbl)
        n204 = local read "平滑"() -> (w352:dbl)
        n205 = call "拼接Z.vi"("Z高频"=w303, "f2"=w251, "Z中频"=w304, "f1"=w252, "Z低频"=w302, "ff"=w301, "f3"=w250) -> ("拼接后Z"=w300:cluster{"X":dbl, "Y":cdb}[])  [unwired: 8 in]
        n206 = for {
          tunnel: w300 -> [w394] mode=indexing
          tunnel: [w393] -> w278 mode=indexing
          tunnel: [w392] -> w282 mode=indexing
          n207 = Unbundle By Name(w394) -> ("X"=w392:dbl, "Y"=w393:cdb)
        }
        n208 = Equal To 0?(x=w352) -> (x = 0?=w275:bool)
        n209 = property on="阻抗Z" class="XYGraph (严格)"("XScale.Maximum"=w250, "XScale.Minimum"=w344, "XScale.Mapping Mode"=w348, "Plot.Plot Color"=w357, "YScale.Mapping Mode"=w348, "YScale.Maximum"=100000.0 ("Y标尺.范围:最大值"), "YScale.Minimum"=1.0 ("Y标尺.范围:最小值")) -> ()  [unwired: 2 in, 2 out]
        n210 = Multiply(x=20.0, y=w358) -> (x*y=w353:dbl)
        n211 = Multiply(x=w352, y=w353) -> (x*y=w265:dbl)
        n212 = Complex To Polar(r * e^(i*theta)=w264) -> (r=w259:dbl[])  [unwired: 1 out]
        n213 = Complex To Re/Im(x + iy=w264) -> (x=w257:dbl[], y=w255:dbl[])
        n214 = Absolute Value(x=w257) -> (abs(x)=w256:dbl[])
        n215 = Absolute Value(x=w255) -> (abs(x)=w254:dbl[])
        n216 = Complex To Re/Im(x + iy=w278) -> (x=w277:dbl[], y=w276:dbl[])
        n217 = Round To Nearest(number=w265) -> (nearest integer value=w266:dbl)
        n218 = Absolute Value(x=w259) -> (abs(x)=w258:dbl[])
        n219 = Absolute Value(x=w276) -> (abs(x)=w270:dbl[])
        n220 = Absolute Value(x=w277) -> (abs(x)=w271:dbl[])
        n221 = Re/Im To Complex(1:w270, 2:w271) -> (0:w272:cdb[])
        n222 = Complex To Polar(r * e^(i*theta)=w272) -> (r=w274:dbl[])  [unwired: 1 out]
        n223 = case shown="假" w275 {
          tunnel: w271 -> [w383 w390]
          tunnel: w270 -> [w381 w389]
          tunnel: w274 -> [w385 w391]
          tunnel: [w384 w391] -> w273
          tunnel: [w382 w390] -> w269
          tunnel: [w380 w389] -> w268
          tunnel: w266 -> [w379 _]
          tunnel: w258 -> [w378 w388]
          tunnel: [w377 w388] -> w263
          tunnel: w256 -> [w376 w387]
          tunnel: [w375 w387] -> w262
          tunnel: w254 -> [w374 w386]
          tunnel: [w373 w386] -> w261
          frame False {
            n224 = call <vilib>:"Median Filter.vi"("right rank"=w379, "left rank"=w379, "X"=w385) -> ("Filtered X"=w384:dbl[])  [unwired: 7 in, 1 out]
            n225 = call <vilib>:"Median Filter.vi"("right rank"=w379, "left rank"=w379, "X"=w383) -> ("Filtered X"=w382:dbl[])  [unwired: 7 in, 1 out]
            n226 = call <vilib>:"Median Filter.vi"("right rank"=w379, "left rank"=w379, "X"=w381) -> ("Filtered X"=w380:dbl[])  [unwired: 7 in, 1 out]
            n227 = call <vilib>:"Median Filter.vi"("right rank"=w379, "left rank"=w379, "X"=w378) -> ("Filtered X"=w377:dbl[])  [unwired: 7 in, 1 out]
            n228 = call <vilib>:"Median Filter.vi"("right rank"=w379, "left rank"=w379, "X"=w376) -> ("Filtered X"=w375:dbl[])  [unwired: 7 in, 1 out]
            n229 = call <vilib>:"Median Filter.vi"("right rank"=w379, "left rank"=w379, "X"=w374) -> ("Filtered X"=w373:dbl[])  [unwired: 7 in, 1 out]
          }
          frame True {
          }
        }
        n230 = Re/Im To Complex(1:w268, 2:w269) -> (0:w267:cdb[])
        n231 = Re/Im To Complex(1:w261, 2:w262) -> (0:w260:cdb[])
        n232 = Bundle By Name(cluster=T3 {"f"=[], "传输阻抗Z"=[], "V"=[], "f_V"=[]} ("吸声测试结果IN"), "f"=w282, "传输阻抗Z"=w267, "V"=w260, "f_V"=w281) -> (w349:T3)
        n233 = Bundle(w282, "Filtered X"=w273) -> (w299:cluster{dbl[], "Filtered X":dbl[]})  [unwired: 1 in]
        n234 = Bundle(w282, "Filtered X"=w269) -> (w298:cluster{dbl[], "Filtered X":dbl[]})  [unwired: 1 in]
        n235 = Bundle(w282, "Filtered X"=w268) -> (w297:cluster{dbl[], "Filtered X":dbl[]})  [unwired: 1 in]
        n236 = Bundle("f"=w281, "Filtered X"=w261) -> (w287:cluster{"f":dbl[], "Filtered X":dbl[]})  [unwired: 1 in]
        n237 = Bundle("f"=w281, "Filtered X"=w263) -> (w285:cluster{"f":dbl[], "Filtered X":dbl[]})  [unwired: 1 in]
        n238 = Bundle("f"=w281, "Filtered X"=w262) -> (w286:cluster{"f":dbl[], "Filtered X":dbl[]})  [unwired: 1 in]
        n239 = Build Array(w285, w286, w287) -> (→"速度V":cluster{"f":dbl[], "Filtered X":dbl[]}[])
        n240 = Build Array(w299, w298, w297) -> (→"阻抗Z":cluster{dbl[], "Filtered X":dbl[]}[])
        n241 = call "Wave Array Record LV2.vi"("吸声测试结果IN"=w349, "W / R"=enum16{"Write", "Read"}."Write") -> ()  [unwired: 1 in, 1 out]
      }
      frame "阻抗管参数设置" {
        n242 = call "parameter setup.vi"() -> ()  [unwired: 12 in]
      }
      frame "输出信号设置" {
        n243 = call "stimulus panel.vi"() -> ("stimulus setup"=→"stimulus setup":T2)  [unwired: 11 in]
      }
      frame "保存测试数据" {
        n244 = flat-sequence {
          frame #0 {
            n245 = local read "阻抗Z"() -> (w429:cluster{dbl[], dbl[]}[])
            n246 = local read "速度V"() -> (w417:cluster{"f":dbl[], dbl[]}[])
            n247 = Index Array(array=w429, index #1=0 ("索引")) -> (element #1=w427:cluster{dbl[], dbl[]}, element #2=w425:cluster{dbl[], dbl[]}, element #3=w426:cluster{dbl[], dbl[]})  [unwired: 2 in]
            n248 = Index Array(array=w417, index #1=0 ("索引")) -> (element #1=w418:cluster{"f":dbl[], dbl[]}, element #2=w420:cluster{"f":dbl[], dbl[]}, element #3=w419:cluster{"f":dbl[], dbl[]})  [unwired: 2 in]
            n249 = Unbundle(w427) -> (w424:dbl[], w423:dbl[])
            n250 = Unbundle(w425) -> (w422:dbl[])  [unwired: 1 out]
            n251 = Unbundle(w426) -> (w421:dbl[])  [unwired: 1 out]
            n252 = Unbundle(w418) -> ("f"=w415:dbl[], w414:dbl[])
            n253 = Unbundle(w420) -> (w413:dbl[])  [unwired: 1 out]
            n254 = Unbundle(w419) -> (w412:dbl[])  [unwired: 1 out]
            n255 = for {
              tunnel: [w451] -> w437 mode=indexing
              tunnel: w424 -> [w450] mode=indexing
              tunnel: w423 -> [w449] mode=indexing
              tunnel: w422 -> [w448] mode=indexing
              tunnel: w421 -> [w447] mode=indexing
              n256 = Number To Fractional String(number=w450) -> (F-format string=w455:string)  [unwired: 3 in]
              n257 = Number To Fractional String(number=w449) -> (F-format string=w454:string)  [unwired: 3 in]
              n258 = Number To Fractional String(number=w447) -> (F-format string=w452:string)  [unwired: 3 in]
              n259 = Number To Fractional String(number=w448) -> (F-format string=w453:string)  [unwired: 3 in]
              n260 = Build Array(w455, w454, w453, w452) -> (w451:string[])
            }
            n261 = for {
              tunnel: [w442] -> w404 mode=indexing
              tunnel: w415 -> [w441] mode=indexing
              tunnel: w414 -> [w440] mode=indexing
              tunnel: w413 -> [w439] mode=indexing
              tunnel: w412 -> [w438] mode=indexing
              n262 = Number To Fractional String(number=w441) -> (F-format string=w446:string)  [unwired: 3 in]
              n263 = Number To Fractional String(number=w440) -> (F-format string=w445:string)  [unwired: 3 in]
              n264 = Number To Fractional String(number=w438) -> (F-format string=w443:string)  [unwired: 3 in]
              n265 = Number To Fractional String(number=w439) -> (F-format string=w444:string)  [unwired: 3 in]
              n266 = Build Array(w446, w445, w444, w443) -> (w442:string[])
            }
            n267 = call <vilib>:"Application Directory.vi"() -> ("Application Directory"=w433:path)
            n268 = call <vilib>:"Application Directory.vi"() -> ("Application Directory"=w408:path)
            n269 = Build Path(base path=w433, name or relative path="传输阻抗Z.csv" ("名称或相对路径")) -> (appended path=w431:path)
            n270 = Build Array (concatenate)(string[] ["f", "Z_abs", "Z_Re", "Z_Im"], w437) -> (w435:string[][])
            n271 = Build Path(base path=w408, name or relative path="流速V.csv" ("名称或相对路径")) -> (appended path=w410:path)
            n272 = Build Array (concatenate)(string[] ["f", "V_abs", "V_Re", "V_Im"], w404) -> (w406:string[][])
            n273 = call-poly <vilib>:"Write Delimited Spreadsheet.vi"("file path (dialog if empty)"=w431, "2D data"=w435, "append to file? (new file:F)"=FALSE, "delimiter (\\t)"="," ("delimiter (\\t)")) -> ()  [unwired: 10 in, 2 out]
            n274 = call-poly <vilib>:"Write Delimited Spreadsheet.vi"("file path (dialog if empty)"=w410, "2D data"=w406, "append to file? (new file:F)"=FALSE, "delimiter (\\t)"="," ("delimiter (\\t)")) -> ()  [unwired: 10 in, 2 out]
          }
          frame #1 {
            n275 = One Button Dialog(message="测试结果已保存" ("消息")) -> ()  [unwired: 1 in, 1 out]
          }
        }
      }
    }
  }
